vi "Read.vi"(8 "error in (no error)":errorcluster, 9 "Variant":variant, 11 "Ethernet in":refnum<class "TCP.lvclass">) -> (0 "error out":errorcluster, 2 "String":string, 3 "Ethernet out":refnum<class "TCP.lvclass">)   [LabVIEW 2013, in "Protocol Classes.lvlib" / "TCP.lvclass"]
uses:
  TCP.lvclass
  Protocol Parent/Methods/Read Parameter.ctl
  TCP.lvclass/TCP.ctl
  Data Access/Read TCP Ref.vi
  Data Access/Write TCP Ref.vi
  Protocol Parent/Protocol Parent.lvclass
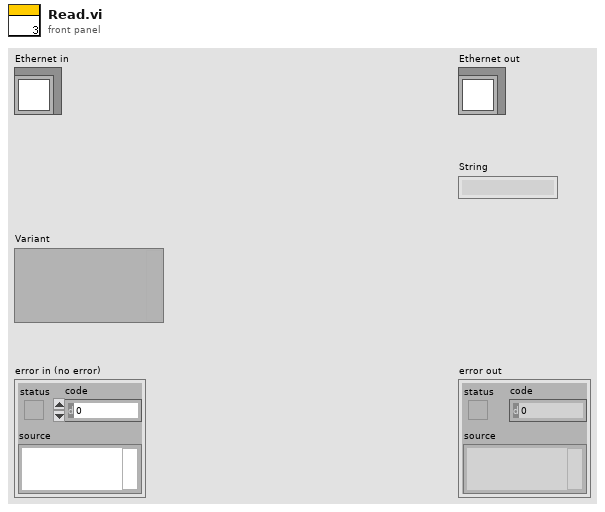
[diagram p1: front panel]
types:
  T1 = typedef "Protocol Classes.lvlib/Protocol Parent.lvclass/Read Parameter.ctl" = cluster{"Wait Type":enum16{"Byte Count", "Wait sec"}, "Wait Value":dbl}
  T2 = enum16{"Standard", "Buffered", "CRLF", "Immediate"}
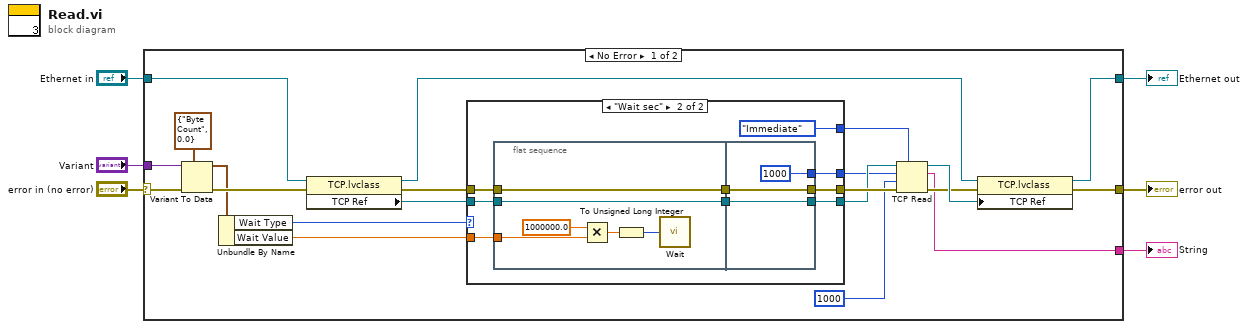
[diagram p0: block diagram]
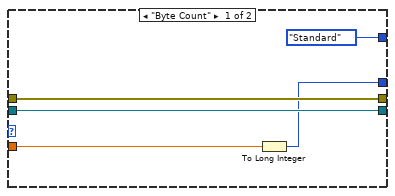
[diagram p2: hidden frame]
diagram:
  n1 = case shown="No Error" "error in (no error)" {
    selector: "error in (no error)" -> [w21 w52]
    tunnel: "Ethernet in" -> [w27 w51]
    tunnel: [w24 w52] -> w3
    tunnel: [w22 w51] -> w2
    tunnel: "Variant" -> [w19 _]
    tunnel: [w10 _] -> w1
    frame No Error {
      n2 = Variant To Data(error in=w21, type=T1 {"Wait Type"=enum."Byte Count", "Wait Value"=0.0} ("Read Parameter"), Variant=w19) -> (data=w18:T1, error out=w20:errorcluster)
      n3 = Unbundle By Name(w18) -> ("Wait Type"=w12:enum16{"Byte Count", "Wait sec"}, "Wait Value"=w11:dbl)
      n4 = property class="TCP.lvclass"(reference=w27, error in=w20) -> (reference out=w23:refnum<class "TCP.lvclass">, error out=w17:errorcluster, "TCP Ref"=w16:refnum<k5>)
      n5 = case shown="\"Wait sec\"" w12 {
        tunnel: w17 -> [w32 w41]
        tunnel: w16 -> [w30 w40]
        tunnel: [w32 w39] -> w15
        tunnel: [w30 w38] -> w14
        tunnel: [w28 w34] -> w13
        tunnel: w11 -> [w31 w35]
        tunnel: [T2."Standard" ("mode (standard)") T2."Immediate" ("mode (standard)")] -> w8
        frame "Byte Count" {
          n6 = To Long Integer(number=w31) -> (32bit integer=w28:i32)
        }
        frame "Wait sec" {
          n7 = flat-sequence {
            tunnel: w40 -> [w46]
            tunnel: w41 -> [w47]
            tunnel: [w47] -> w37
            tunnel: [w46] -> w36
            tunnel: w35 -> [w45]
            tunnel: [w50] -> w39
            tunnel: [w49] -> w38
            tunnel: w37 -> [w50]
            tunnel: w36 -> [w49]
            tunnel: [1000 ("Wait Value")] -> w34
            frame #0 {
              n8 = Multiply(x=1000000.0, y=w45) -> (x*y=w44:dbl)
              n9 = To Unsigned Long Integer(number=w44) -> (unsigned 32bit integer=w42:u32)
              n10 = call "Wait"("Count(uSec)"=w42) -> ()  [unwired: 1 out]
            }
            frame #1 {
            }
          }
        }
      }
      n11 = TCP Read(connection ID=w14, bytes to read=w13, error in (no error)=w15, 7:w8, 9:1000 ("timeout ms (25000)")) -> (connection ID out=w26:refnum<k5>, data out=w10:string, error out=w25:errorcluster)
      n12 = property class="TCP.lvclass"(reference=w23, error in=w25, "TCP Ref"=w26) -> (reference out=w22:refnum<class "TCP.lvclass">, error out=w24:errorcluster)
    }
    frame Error {
    }
  }
  "error out" <- w3
  "Ethernet out" <- w2
  "String" <- w1
